vi "Write Control Metadata.vi"(8 "error in":errorcluster, 10 "control metadata":T1={"Limit Low"=variant(dbl 0.0), "Limit High"=variant(dbl 0.0), "Min Step"=variant(dbl 0.0)}, 11 "PV Data in":refnum<class "PV Data.lvclass">) -> (0 "error out":errorcluster, 3 "PV Data out":refnum<class "PV Data.lvclass">)   [LabVIEW 2020, in "PV Access.lvlib" / "PV Data.lvlib" / "PV Data.lvclass"]
uses:
  PV Data.lvclass
  2d83a253-f0d6-4305-b049-10d4b2f93fa3.vi
  c9cbd3a0-b478-4a5c-977b-556fdc0fb382.vi
  51f27453-05f5-4ccc-a431-2c551ab4ec3d.vi
  Control Metadata.ctl
  PV Data.lvlib
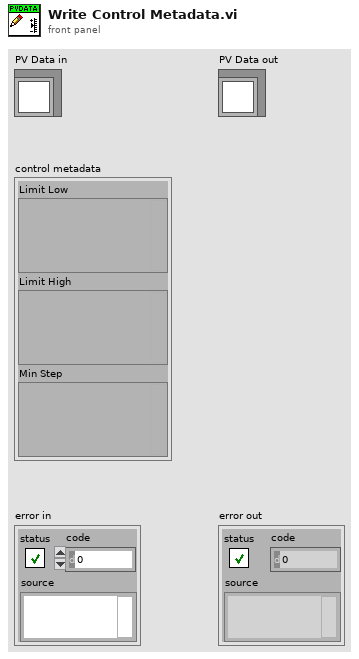
[diagram p1: front panel]
types:
  T1 = typedef "PV Access.lvlib/PV Data.lvlib/Control Metadata.ctl" = cluster{"Limit Low":variant, "Limit High":variant, "Min Step":variant}
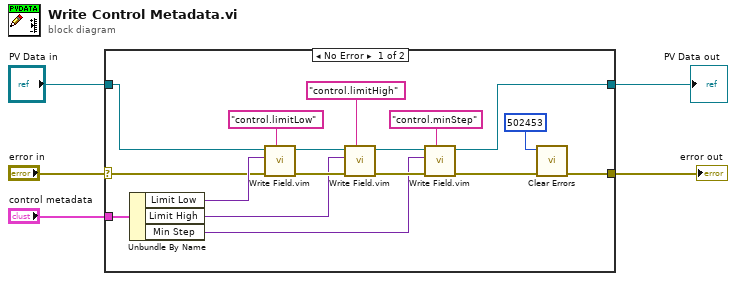
[diagram p0: block diagram]
diagram:
  n1 = case shown="No Error" "error in" {
    selector: "error in" -> [w12 w24]
    tunnel: [w6 w24] -> w3
    tunnel: "PV Data in" -> [w11 w23]
    tunnel: [w8 w23] -> w5
    tunnel: "control metadata" -> [w10 _]
    frame No Error {
      n2 = Unbundle By Name(w10) -> ("Limit Low"=w15:variant, "Limit High"=w13:variant, "Min Step"=w14:variant)
      n3 = call "Write Field.vim"("field name"="control.limitLow", "error in"=w12, "value in"=w15, "PV Data in"=w11) -> ("error out"=w22:errorcluster, "PV Data out"=w19:refnum<class "PV Data.lvclass">)  [unwired: 5 in, 1 out]
      n4 = call "Write Field.vim"("field name"="control.limitHigh", "error in"=w22, "value in"=w13, "PV Data in"=w19) -> ("error out"=w21:errorcluster, "PV Data out"=w20:refnum<class "PV Data.lvclass">)  [unwired: 5 in, 1 out]
      n5 = call "Write Field.vim"("field name"="control.minStep", "error in"=w21, "value in"=w14, "PV Data in"=w20) -> ("error out"=w7:errorcluster, "PV Data out"=w8:refnum<class "PV Data.lvclass">)  [unwired: 5 in, 1 out]
      n6 = call <vilib>:"Clear Errors.vi"("error in (no error)"=w7, "specific error code to clear (0: all)"=502453) -> ("error out"=w6:errorcluster)  [unwired: 4 in, 1 out]
    }
    frame Error {
    }
  }
  "error out" <- w3
  "PV Data out" <- w5
